vi "Digio Write Bit.vi"(5 "Data (0)":u32 max=1, 7 "Bit (1)":u32=1 min=1 max=14, 8 "error in (no error)":errorcluster, 10 "Node In":string, 11 "VISA resource name":refnum<visa-resource-name>) -> (0 "error out":errorcluster, 2 "Node Out":string, 3 "VISA resource name out":refnum<visa-resource-name>, 4 "Command String":string)   [LabVIEW 2012, in "Keithley 2600 Series.lvlib"]
doc: "This VI will set a digital I/O line high or low.\n\nIf the output line is write protected, via the digio.writeprotect attribute, the command will be ignored.\n\nThe reset function does not affect the present states of the digital I/O lines.\n\n<b>Functions and Attributes Used</b>\ndigio.writebit(bit, data)\nbit = Digital I/O line number (1 to 14)\ndata = Value to write to the bit; 0 (low) or 1 (high)\n\nNote:\nDigital IO feature is not supported with Keithley 2604B, 2614B, 2634B."
uses:
  Keithley 2600 Series.lvlib
  Private/GlobalVariables.vi
panel:
  # "(c) 2008 Keithley Instruments, Inc.  ALL RIGHTS RESERVED."
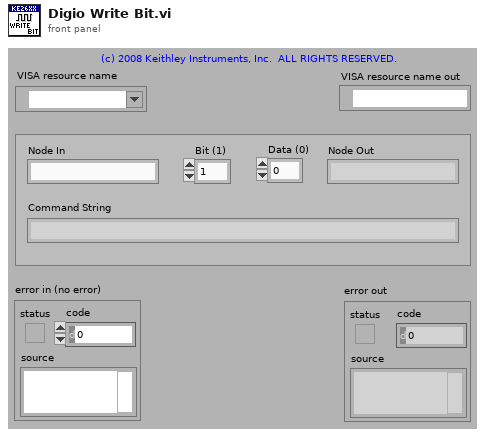
[diagram p1: front panel]
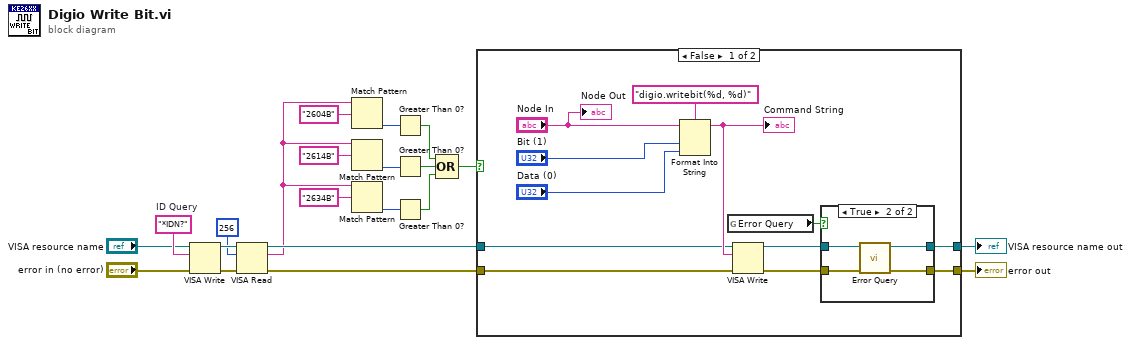
[diagram p0: block diagram]
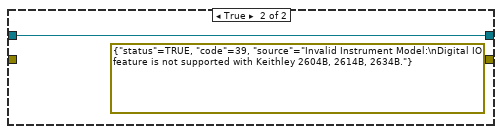
[diagram p3: hidden frame]
diagram:
  w16 = "*IDN?"  # ID Query
  n1 = VISA Write(VISA resource name="VISA resource name", write buffer=w16, error in (no error)="error in (no error)") -> (VISA resource name out=w19:refnum<visa-resource-name>, error out=w18:errorcluster)  [unwired: 1 out]
  n2 = VISA Read(VISA resource name=w19, byte count=u32 256, error in (no error)=w18) -> (VISA resource name out=w15:refnum<visa-resource-name>, read buffer=w1:string, error out=w14:errorcluster)  [unwired: 1 out]
  n3 = Match Pattern(string=w1, regular expression="2604B" ("y")) -> (offset past match=w8:i32)  [unwired: 1 in, 3 out]
  n4 = Match Pattern(string=w1, regular expression="2614B" ("y")) -> (offset past match=w7:i32)  [unwired: 1 in, 3 out]
  n5 = Match Pattern(string=w1, regular expression="2634B" ("y")) -> (offset past match=w6:i32)  [unwired: 1 in, 3 out]
  n6 = Greater Than 0?(x=w8) -> (x > 0?=w5:bool)
  n7 = Greater Than 0?(x=w7) -> (x > 0?=w4:bool)
  n8 = Greater Than 0?(x=w6) -> (x > 0?=w3:bool)
  n9 = Compound Arithmetic op=OR(w5, w4, w3) -> (w2:bool)
  n10 = case shown="False" w2 {
    tunnel: [w30 w41] -> w21
    tunnel: [w29 errorcluster {"status"=TRUE, "code"=39, "source"="Invalid Instrument Model:\nDigital IO feature is not supported with Keithley 2604B, 2614B, 2634B."} ("error out")] -> w20
    tunnel: w15 -> [w23 w41]
    tunnel: w14 -> [w22 _]
    frame False {
      n11 = Format Into String(format string="digio.writebit(%d, %d)", initial string="Node In", "Bit (1)", "Data (0)") -> (resulting string=w24:string)  [unwired: 1 in, 1 out]
      "Command String" <- w24
      n12 = global read "GlobalVariables.vi" "Error Query"() -> (w33:bool)
      n13 = VISA Write(VISA resource name=w23, write buffer=w24, error in (no error)=w22) -> (VISA resource name out=w32:refnum<visa-resource-name>, error out=w31:errorcluster)  [unwired: 1 out]
      n14 = case shown="True" w33 {
        tunnel: w32 -> [w35 w39]
        tunnel: w31 -> [w34 w38]
        tunnel: [w35 w37] -> w30
        tunnel: [w34 w36] -> w29
        frame False {
        }
        frame True {
          n15 = call "Error Query.vi"("error in (no error)"=w38, "VISA resource name"=w39) -> ("error out"=w36:errorcluster, "VISA resource name out"=w37:refnum<visa-resource-name>)  [unwired: 8 out]
        }
      }
      "Node Out" <- "Node In"
    }
    frame True {
    }
  }
  "VISA resource name out" <- w21
  "error out" <- w20
